vi "CheckResponse.vi"(8 "error in":errorcluster {"code" format="%.0x"}, 10 "SID":u8 format="%02x", 11 "DataIn":u8[](array[numeric]) format="%02x") -> (0 "error out":errorcluster, 3 "DataOut":u8[](array[numeric]) format="%02x")   [LabVIEW 2011, in "Konvolucio MUDS150628.lvlib"]
uses:
  <instrlib>/Konvolucio MUDS150628/Konvolucio MUDS150628.lvlib
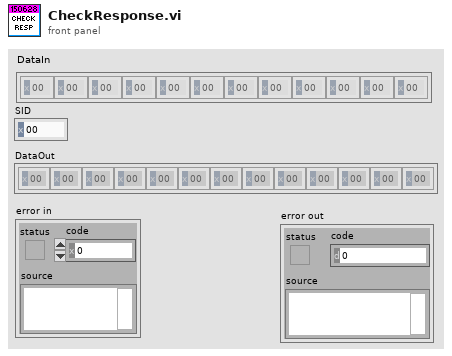
[diagram p1: front panel]
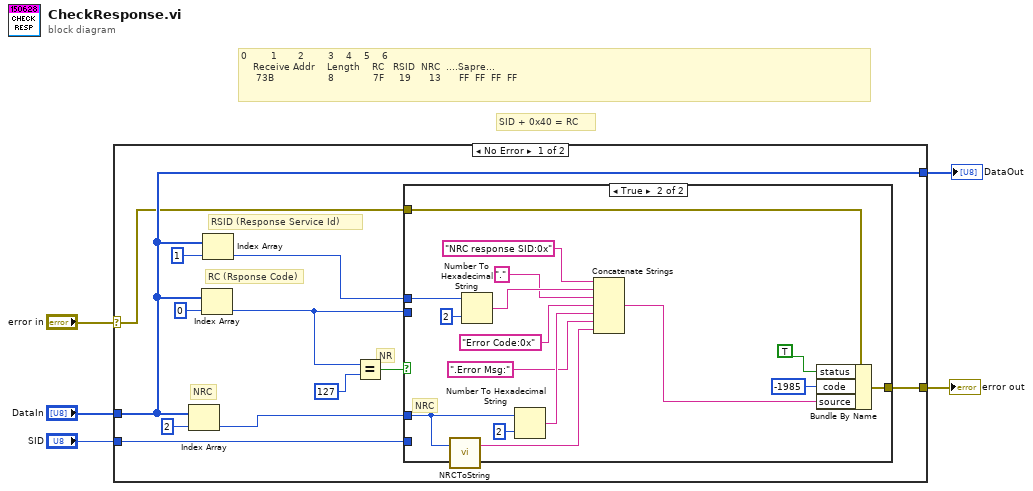
[diagram p0: block diagram]
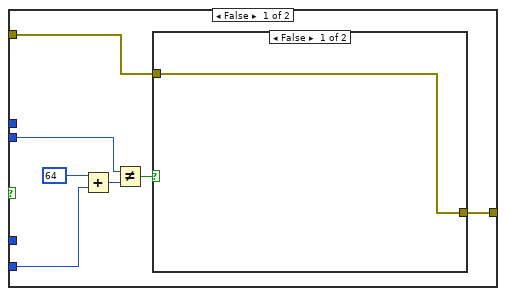
[diagram p2: hidden frame]
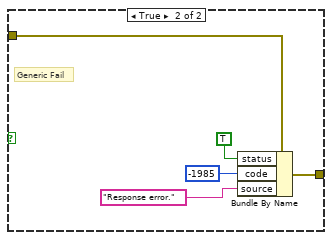
[diagram p3: hidden frame]
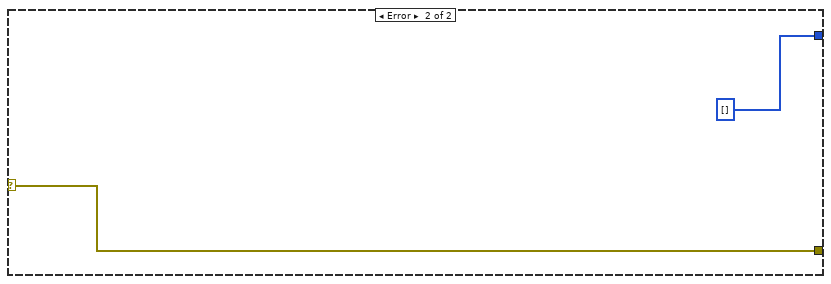
[diagram p4: hidden frame]
diagram:
  # "SID + 0x40 = RC"
  # "0        1       2        3    4    5    6  \n    Receive Addr    Length    RC   RSID  NRC  ....Sapre...\n     73B                  8             7F     19      13      FF  FF  FF  FF"
  n1 = case shown="No Error" "error in" {
    selector: "error in" -> [w6 w47]
    tunnel: [w7 w47] -> w1
    tunnel: "DataIn" -> [w10 _]
    tunnel: "SID" -> [w8 _]
    tunnel: [w10 u8[] [] ("DataIn")] -> w2
    frame No Error {
      # "NRC"
      # "RSID (Response Service Id)"
      # "NR"
      # "RC (Rsponse Code)"
      n2 = Index Array(array=w10, index=2) -> (element=w12:u8)
      n3 = Index Array(array=w10, index=0) -> (element=w9:u8)
      n4 = Index Array(array=w10, index=1) -> (element=w14:u8)
      n5 = Equal?(x=w9, y=u8 127 ("Init")) -> (x = y?=w11:bool)
      n6 = case shown="True" w11 {
        tunnel: w12 -> [_ w31]
        tunnel: w14 -> [_ w46]
        tunnel: [w18 w34] -> w7
        tunnel: w6 -> [w19 w33]
        tunnel: w9 -> [w23 _]
        tunnel: w8 -> [w20 _]
        frame False {
          n7 = Add(x=u8 64, y=w20) -> (x+y=w24:u8)
          n8 = Not Equal?(x=w23, y=w24) -> (x != y?=w22:bool)
          n9 = case shown="False" w22 {
            tunnel: [w25 w27] -> w18
            tunnel: w19 -> [w25 w26]
            frame False {
            }
            frame True {
              # "Generic Fail"
              n10 = Bundle By Name(cluster=w26, "status"=TRUE, "code"=-1985, "source"="Response error." ("string")) -> (w27:errorcluster)
            }
          }
        }
        frame True {
          # "NRC"
          n11 = call <instrlib>:"NRCToString.vi"("SIDRQ"=w31) -> ("NRC Message"=w32:string)  [unwired: 2 in]
          n12 = Number To Hexadecimal String(1:i16 2 ("width (-)"), 2:w46) -> (0:w43:string)
          n13 = Number To Hexadecimal String(1:i16 2 ("width (-)"), 2:w31) -> (0:w39:string)
          n14 = Concatenate Strings("NRC response SID:0x" ("string"), w43, "." ("string"), "Error Code:0x" ("string"), w39, ".Error Msg:" ("string"), w32) -> (w35:string)
          n15 = Bundle By Name(cluster=w33, "status"=TRUE, "code"=-1985, "source"=w35) -> (w34:errorcluster)
        }
      }
    }
    frame Error {
    }
  }
  "error out" <- w1
  "DataOut" <- w2
